vi "Savitsky Golay Weighted Filter.vi"   [LabVIEW 2019, in "xy_utilities.lvlib"]
doc: "Filter <b>XY-data</b>'s Y-Array with a Savitsky-Golay FIR smoothing filter.\n\n<b>side points</b> specifies the number of data points to each side of the current data point to use for the least squares minimization. side points*2 + 1 is the length of the moving window, which must be greater than the polynomial order.\n\n<b>polynomial order</b> specifies the order of the polynomial. \n\nWire data to the data input to determine the polymorphic instance to use or manually select the instance."
uses:
  xy_utilities.lvlib
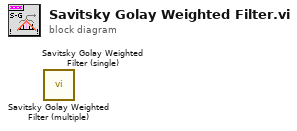
[diagram p0: block diagram]
diagram:
  n1 = call "Savitsky Golay Weighted Filter (multiple).vi"() -> ()  [unwired: 10 in, 2 out]
  n2 = call "Savitsky Golay Weighted Filter (single).vi"() -> ()  [unwired: 10 in, 2 out]
